vi "FA_ApplyShared Variables.vi"(8 "Error In":errorcluster) -> (0 "Error Out":errorcluster)   [LabVIEW 2014, in "FA_SharedVariables.lvlib"]
doc: "Reads the general XML config data from file, formats the shared variable data, and writes the XML result to file"
uses:
  FA_SharedVariables.lvlib
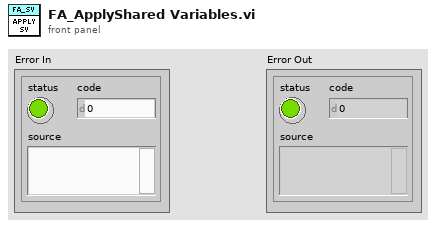
[diagram p1: front panel]
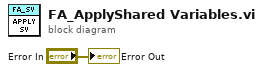
[diagram p0: block diagram]
diagram:
  "Error Out" <- "Error In"
